vi "InsertNode.vi"(9 "KD-Tree":T1=[{"axis"=enum."x", "value"=5.0, "left"=inf, "right"=inf, "Point"=[1.0, 5.0, 25.0, 0.0]}], 10 "New Node":dbl[](array[numeric])) -> (2 "New KD-Tree":T1)   [LabVIEW 2023]
uses:
  KD-Tree.ctl
  Node.ctl
panel:
  in  "index":i32
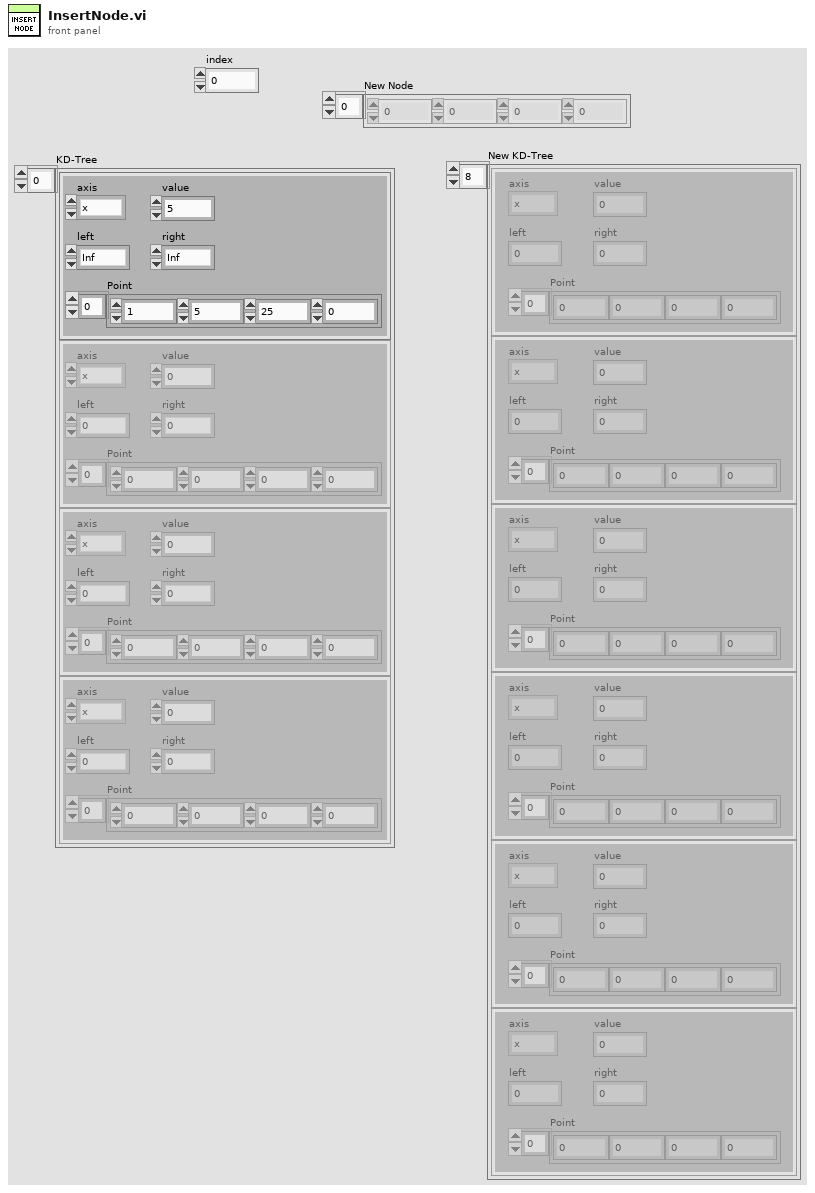
[diagram p1: front panel]
types:
  T1 = typedef "KD-Tree.ctl" = T2[]
  T2 = typedef "Node.ctl" = cluster{"axis":enum16{"null", "x", "y"}, "value":dbl, "left":dbl, "right":dbl, "Point":dbl[]}
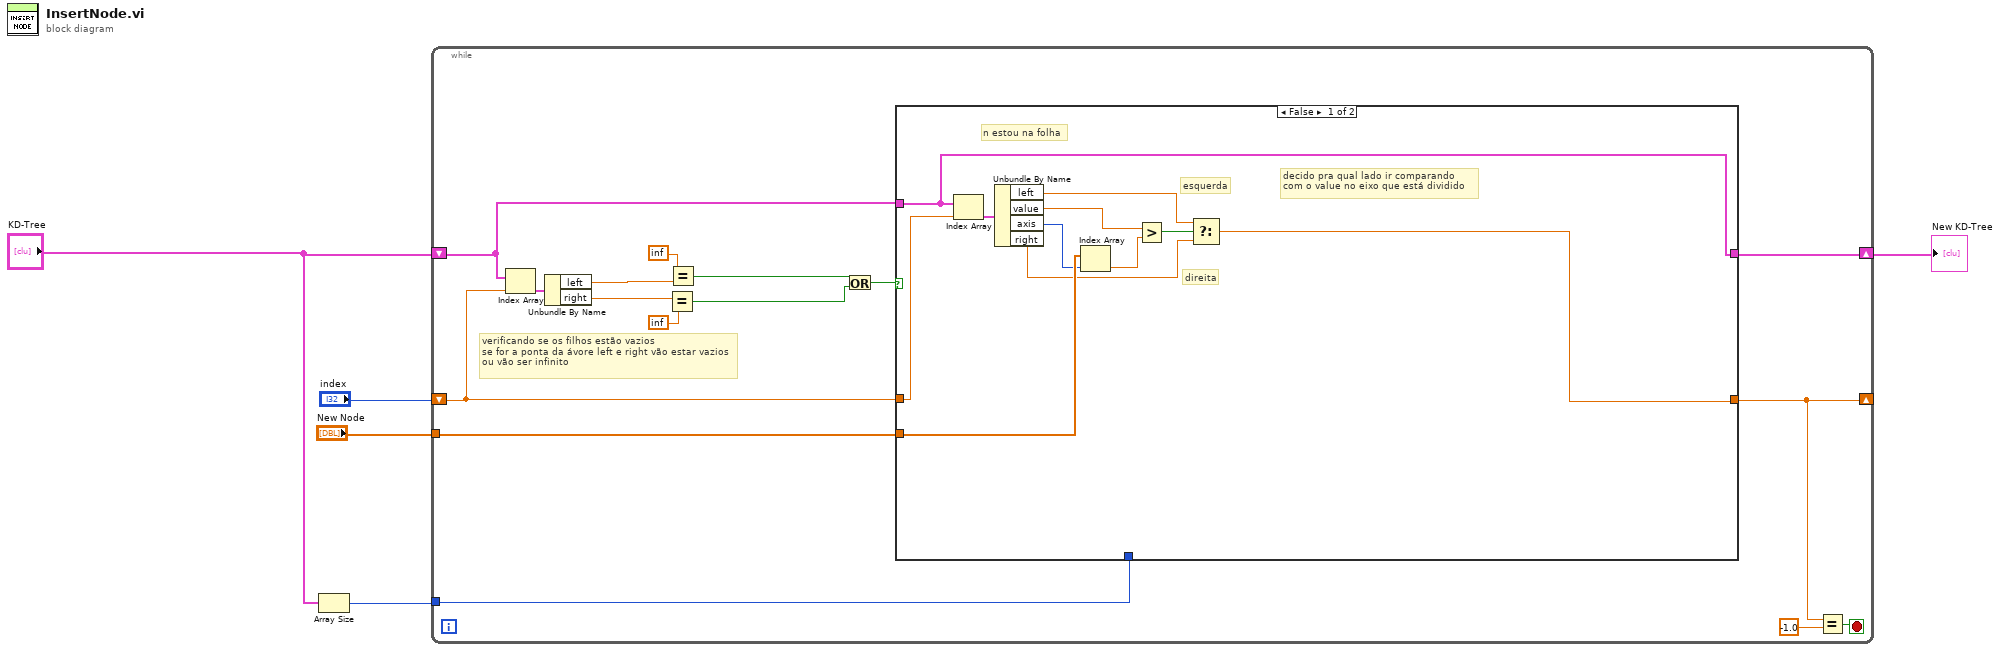
[diagram p0: block diagram]
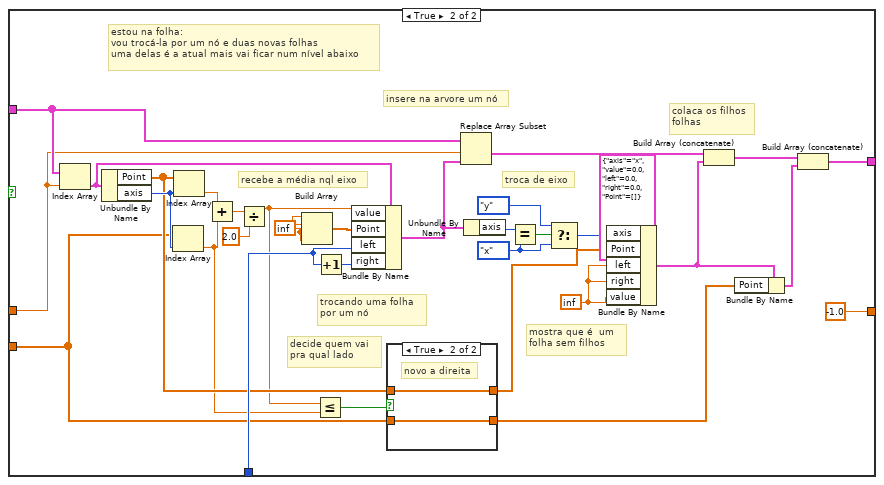
[diagram p2: hidden frame]
diagram:
  n1 = Array Size(array="KD-Tree") -> (size(s)=w4:i32)
  n2 = while {
    tunnel: w4 -> [w18]
    tunnel: "New Node" -> [w14]
    shift-right: [w9] -> w1
    shift-left: "KD-Tree" -> [w17]
    shift-right: [w6] -> _
    shift-left: "index" -> [w20]
    stop <- w8 stop-if-true
    # "verificando se os filhos estão vazios\nse for a ponta da ávore left e right vão estar vazios\nou vão ser infinito"
    n3 = Index Array(array=w17, index=w20) -> (element=w19:T2)
    n4 = Unbundle By Name(w19) -> ("left"=w12:dbl, "right"=w13:dbl)
    n5 = Equal?(x=w13, y=inf) -> (x = y?=w10:bool)
    n6 = Equal?(x=inf, y=w12) -> (x = y?=w11:bool)
    n7 = Or(x=w11, y=w10) -> (x .or. y?=w16:bool)
    n8 = case shown="False" w16 {
      tunnel: w17 -> [w22 w63]
      tunnel: w20 -> [w31 w58]
      tunnel: w18 -> [_ w54]
      tunnel: w14 -> [w30 w40]
      tunnel: [w22 w44] -> w9
      tunnel: [w23 -1.0] -> w6
      frame False {
        # "decido pra qual lado ir comparando \ncom o value no eixo que está dividido"
        # "n estou na folha"
        # "direita"
        # "esquerda"
        n9 = Index Array(array=w22, index=w31) -> (element=w32:T2)
        n10 = Unbundle By Name(w32) -> ("left"=w25:dbl, "value"=w26:dbl, "axis"=w29:enum16{"null", "x", "y"}, "right"=w24:dbl)
        n11 = Index Array(array=w30, index=w29) -> (element=w28:dbl)
        n12 = Greater?(x=w26, y=w28) -> (0:w27:bool)
        n13 = Select(t=w25, s=w27, f=w24) -> (s? t:f=w23:dbl)
      }
      frame True {
        w47 = inf
        w49 = enum16{"null", "x", "y"}."x" ("y")
        w34 = inf
        # "estou na folha:\nvou trocá-la por um nó e duas novas folhas \numa delas é a atual mais vai ficar num nível abaixo"
        # "decide quem vai \npra qual lado"
        # "mostra que é  um \nfolha sem filhos"
        # "troca de eixo"
        # "recebe a média nql eixo"
        # "trocando uma folha\npor um nó"
        # "insere na arvore um nó"
        # "colaca os filhos\nfolhas"
        n14 = Index Array(array=w63, index=w58) -> (element=w57:T2)
        n15 = Unbundle By Name(w57) -> ("Point"=w41:dbl[], "axis"=w62:enum16{"null", "x", "y"})
        n16 = Index Array(array=w40, index=w62) -> (element=w39:dbl)
        n17 = Index Array(array=w41, index=w62) -> (element=w61:dbl)
        n18 = Add(x=w61, y=w39) -> (x+y=w60:dbl)
        n19 = Divide(x=w60, y=2.0) -> (x/y=w33:dbl)
        n20 = Build Array(w34, w34, w34, w34) -> (w56:dbl[])
        n21 = Less Or Equal?(x=w33, y=w39) -> (x <= y?=w38:bool)
        n22 = Increment(x=w54) -> (x+1=w55:i32)
        n23 = Bundle By Name(cluster=w57, "value"=w33, "Point"=w56, "left"=w54, "right"=w55) -> (w53:T2)
        n24 = case shown="True" w38 {
          tunnel: w41 -> [w65 w67]
          tunnel: w40 -> [w66 w68]
          tunnel: [w65 w68] -> w37
          tunnel: [w66 w67] -> w36
          frame False {
            # "novo a esquerda"
          }
          frame True {
            # "novo a direita"
          }
        }
        n25 = Replace Array Subset(array=w63, new element=w53, index=w58) -> (w46:T1)
        n26 = Unbundle By Name(w53) -> ("axis"=w51:enum16{"null", "x", "y"})
        n27 = Equal?(x=w51, y=w49) -> (x = y?=w52:bool)
        n28 = Select(t=enum16{"null", "x", "y"}."y" ("y"), s=w52, f=w49) -> (s? t:f=w48:enum16{"null", "x", "y"})
        n29 = Bundle By Name(cluster=T2 {"axis"=enum."x", "value"=0.0, "left"=0.0, "right"=0.0, "Point"=[]} ("Node 2"), "axis"=w48, "Point"=w36, "left"=w47, "right"=w47, "value"=w47) -> (w43:T2)
        n30 = Build Array (concatenate)(w46, w43) -> (w45:T1)
        n31 = Bundle By Name(cluster=w43, "Point"=w37) -> (w42:T2)
        n32 = Build Array (concatenate)(w45, w42) -> (w44:T1)
      }
    }
    n33 = Equal?(x=w6, y=-1.0) -> (x = y?=w8:bool)
  }
  "New KD-Tree" <- w1
